vi "data std sequence 17O Simple.vi"(8 "error in":errorcluster) -> (3 "cycle results cluster out":T1, 11 "cycle results cluster IN":T1)   [LabVIEW 2016]
doc: "Takes a sample type and sorts by sequence"
uses:
  controls/cycle results control.ctl
  <vilib>/Analysis/baseanly.llb/Mean (DBL).vi
  <vilib>/Analysis/NI_AALBase.lvlib
panel:
  out "error out":errorcluster
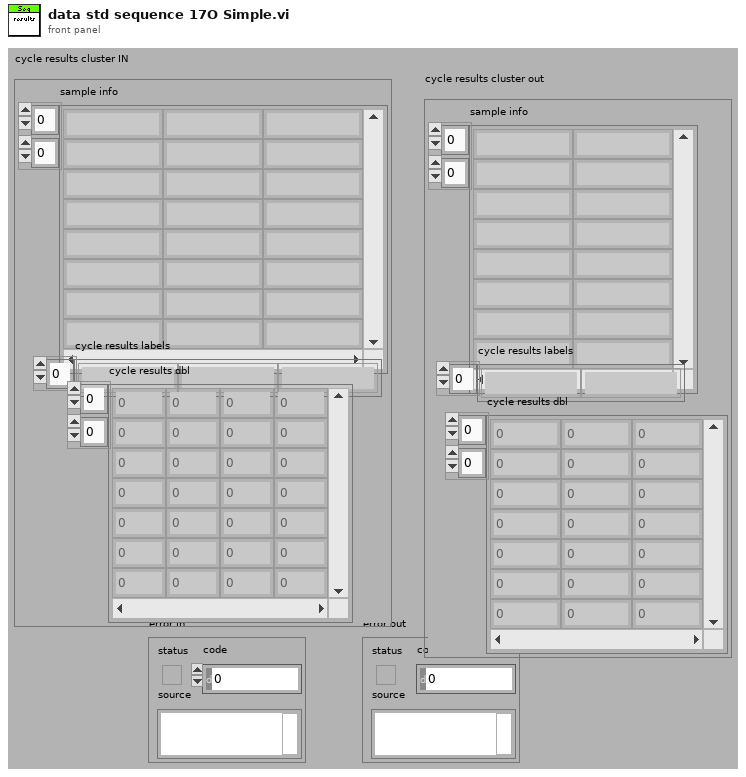
[diagram p1: front panel]
types:
  T1 = typedef "cycle results control.ctl" = cluster{"sample info":string[][], "cycle results labels":string[], "cycle results dbl":dbl[][]}
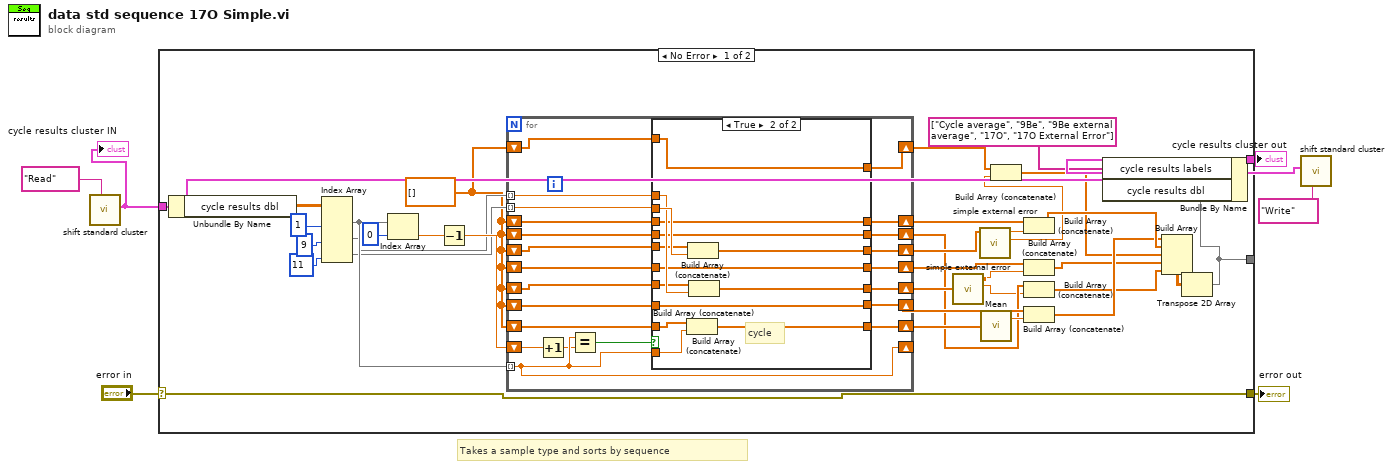
[diagram p0: block diagram]
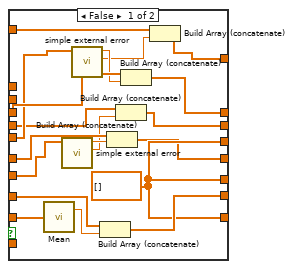
[diagram p2: hidden frame]
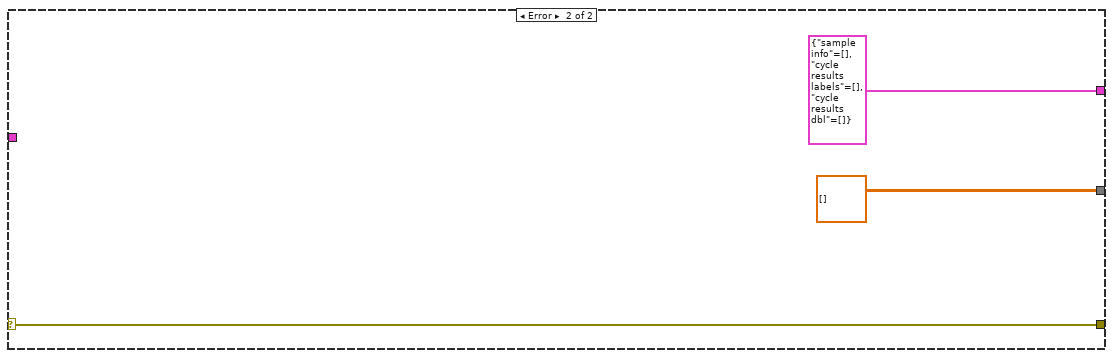
[diagram p3: hidden frame]
diagram:
  # "Takes a sample type and sorts by sequence"
  n1 = call "shift standard cluster.vi"("read write shift"="Read") -> ("cycle results cluster out"=w1:T1)  [unwired: 9 in, 1 out]
  "cycle results cluster IN" <- w1
  n2 = case shown="No Error" "error in" {
    selector: "error in" -> [w24 w98]
    tunnel: w1 -> [w23 _]
    tunnel: [w19 dbl[][] []] -> _
    tunnel: [w21 T1 {"sample info"=[], "cycle results labels"=[], "cycle results dbl"=[]} ("cycle results cluster IN")] -> w3
    tunnel: [w24 w98] -> w5
    frame No Error {
      w7 = dbl[] []
      n3 = Unbundle By Name(w23) -> ("cycle results dbl"=w33:dbl[][])
      n4 = Index Array(array=w33, index (col) #1=1 ("disabled index (col)"), index (col) #2=9 ("index (col)"), index (col) #3=11 ("index (col)")) -> (element #1=w29:dbl[], element #2=w28:dbl[], element #3=w27:dbl[])  [unwired: 3 in]
      n5 = Index Array(array=w29, index=0) -> (element=w36:dbl)
      n6 = Decrement(x=w36) -> (x-1=w35:dbl)
      n7 = for {
        tunnel: w29 -> [w57] mode=indexing
        shift-right: [w61] -> w37
        shift-left: w7 -> [w60]
        shift-right: [w59] -> w41
        shift-left: w7 -> [w58]
        shift-right: [w57] -> _
        shift-left: w35 -> [w63]
        tunnel: w27 -> [w56] mode=indexing
        tunnel: w28 -> [w55] mode=indexing
        shift-right: [w54] -> w14
        shift-left: w7 -> [w51]
        shift-right: [w53] -> w18
        shift-left: w7 -> [w52]
        shift-right: [w50] -> w38
        shift-left: w7 -> [w48]
        shift-right: [w49] -> w39
        shift-left: w7 -> [w47]
        shift-right: [w45] -> w15
        shift-left: w7 -> [w44]
        shift-right: [w43] -> w12
        shift-left: w7 -> [w42]
        n8 = Increment(x=w63) -> (x+1=w46:dbl)
        n9 = Equal?(x=w57, y=w46) -> (x = y?=w62:bool)
        n10 = case shown="True" w62 {
          tunnel: w57 -> [_ w93]
          tunnel: [w78 w96] -> w61
          tunnel: w60 -> [w82 w94]
          tunnel: [w81 w95] -> w59
          tunnel: w58 -> [w80 w95]
          tunnel: w56 -> [_ w92]
          tunnel: w55 -> [_ w91]
          tunnel: [w78 w90] -> w54
          tunnel: [w78 w89] -> w53
          tunnel: w52 -> [w70 w88]
          tunnel: w51 -> [w68 w87]
          tunnel: [w77 w86] -> w50
          tunnel: [w76 w85] -> w49
          tunnel: w48 -> [w75 w86]
          tunnel: w47 -> [w74 w85]
          tunnel: [w73 w84] -> w45
          tunnel: w44 -> [w72 w84]
          tunnel: [w65 w83] -> w43
          tunnel: w42 -> [w64 w83]
          frame False {
            w78 = dbl[] []
            n11 = call-poly <vilib>:"Mean.vi"("X"=w82) -> ("mean"=w79:dbl)  [unwired: 1 out]
            n12 = call "simple external error.vi"("cycle results"=w68) -> ("External error"=w66:dbl, "Sequence result"=w67:dbl)  [unwired: 7 in, 2 out]
            n13 = call "simple external error.vi"("cycle results"=w70) -> ("External error"=w69:dbl, "Sequence result"=w71:dbl)  [unwired: 7 in, 2 out]
            n14 = Build Array (concatenate)(w80, w79) -> (w81:dbl[])
            n15 = Build Array (concatenate)(w74, w67) -> (w76:dbl[])
            n16 = Build Array (concatenate)(w64, w66) -> (w65:dbl[])
            n17 = Build Array (concatenate)(w75, w71) -> (w77:dbl[])
            n18 = Build Array (concatenate)(w72, w69) -> (w73:dbl[])
          }
          frame True {
            # "cycle"
            n19 = Build Array (concatenate)(w94, w93) -> (w96:dbl[])
            n20 = Build Array (concatenate)(w88, w92) -> (w89:dbl[])
            n21 = Build Array (concatenate)(w87, w91) -> (w90:dbl[])
          }
        }
      }
      n22 = call "simple external error.vi"("cycle results"=w14) -> ("External error"=w11:dbl, "Sequence result"=w13:dbl)  [unwired: 7 in, 2 out]
      n23 = call "simple external error.vi"("cycle results"=w18) -> ("External error"=w16:dbl, "Sequence result"=w17:dbl)  [unwired: 7 in, 2 out]
      n24 = call-poly <vilib>:"Mean.vi"("X"=w37) -> ("mean"=w40:dbl)  [unwired: 1 out]
      n25 = Build Array (concatenate)(w15, w16) -> (w10:dbl[])
      n26 = Build Array (concatenate)(w38, w17) -> (w26:dbl[])
      n27 = Build Array (concatenate)(w39, w13) -> (w9:dbl[])
      n28 = Build Array (concatenate)(w12, w11) -> (w8:dbl[])
      n29 = Build Array (concatenate)(w41, w40) -> (w25:dbl[])
      n30 = Build Array(w25, w26, w10, w9, w8) -> (w20:dbl[][])
      n31 = Transpose 2D Array(2D array=w20) -> (transposed array=w19:dbl[][])
      n32 = Bundle By Name(cluster=w23, "cycle results labels"=string[] ["Cycle average", "9Be", "9Be external average", "17O", "17O External Error"], "cycle results dbl"=w19) -> (w21:T1)
    }
    frame Error {
    }
  }
  "error out" <- w5
  "cycle results cluster out" <- w3
  n33 = call "shift standard cluster.vi"("read write shift"="Write", "cycle results cluster In"=w3) -> ()  [unwired: 8 in, 2 out]
